vi "pulse_detector_usrp_implemented.vi"() -> ()   [LabVIEW 2021]
doc: "Acquires data from the Rx ports and streams the data to the host while receiving data from the host and generating the resulting waveform at the Tx ports of the NI USRP-294x/295x device. Use this VI as a template for the Simple NI-USRP Streaming sample project."
uses:
  <instrlib>/_niInstr/Register Bus/v1/FPGA/Public/Read Cmd Data.ctl
  SubVIs/Tx Parameters.ctl
  Host/SubVIs/Start Trigger.ctl
  SubVIs/DUC Parameters.ctl
  <instrlib>/_niInstr/DSP/v1/Shared/Public/IQ Impairments.ctl
  <instrlib>/_niInstr/DSP/v1/Shared/Public/IQ Gain.ctl
  SubVIs/Stream Control State.ctl
  SubVIs/Rx Parameters.ctl
  SubVIs/DDC Parameters.ctl
  reciver params.ctl
  <vilib>/Platform/TimedLoop/XDataNode/timing_clust.ctl
  <vilib>/Platform/TimedLoop/XDataNode/nitl_modes.ctl
  <vilib>/Platform/TimedLoop/XDataNode/wakeup.ctl
  <vilib>/rvi/Emulation/niFpgaSctlEmulationGetInTimedLoop.vi
  <vilib>/rvi/Emulation/niFpgaEmulationReportErrorSimple.vi
  <vilib>/rvi/Emulation/niFpgaGetClockAttributes.vi
  <vilib>/rvi/Emulation/niFpgaCriticalErrorInLSC.vi
  <vilib>/rvi/Emulation/niFpgaProcessEmulError.vi
  <vilib>/rvi/eio/common/nirviEmuTemplateMethod_errors.vi
  <vilib>/rvi/interface/RandomDataEmulation/niFpgaRandomDataHandleErrors.vi
  <vilib>/Platform/TimedLoop/XDataNode/XDataNode.xnode
  <vilib>/eio/EIONode/EIONode.xnode
  <vilib>/rvi/DataTransferAndStorage/Container/XNode/niFpgaContainer.xnode
  <vilib>/rvi/interface/RandomDataEmulation/nirviRandomDataFpgaReadWriteTemplate.vi
  <vilib>/Platform/TimedLoop/XDataNode/XDNodeRunTimeDep.lvlib
  <instrlib>/_niInstr/Register Bus/v1/FPGA/niInstr Register Bus v1 FPGA.lvlib
  <instrlib>/niUsrpRio/Config/v1/FPGA/niUsrpRio Config v1 FPGA.lvlib
  <instrlib>/_niInstr/DSP/v1/Shared/niInstr DSP v1 Shared.lvlib
panel:
  in  "reciver_params":T1
  in  "rx 3.led":T2(ring)
  in  "rx 2.led":T2(ring)
  in  "rx 0.led":T2(ring)
  in  "rx 1.led":T2(ring)
  in  "tx 0.led":enum16{"None", "RF 0/TX 1", "RF 1/TX 1"}(ring)
  in  "tx 1.led":enum16{"None", "RF 0/TX 1", "RF 1/TX 1"}(ring)
  in  "rx 3.stream enable":bool
  in  "rx 2.stream enable":bool
  out "rx 3.number of iq data overflows":u64
  out "rx 2.number of iq data overflows":u64
  in  "rx 3.phase":fxp<+/-,21,0>
  in  "rx 3.frequency shift":fxp<+/-,48,0> format="%#.48g"
  in  "rx 3.impairments":T3={"inline gain I"=0.9999923706054688, "inline gain Q"=0.9999923706054688, "cross gain I"=0.0, "cross gain Q"=0.0, "pre-gain offset I"=0.0, "pre-gain offset Q"=0.0, "post-gain offset I"=0.0, "post-gain offset Q"=0.0}
  in  "rx 2.phase":fxp<+/-,21,0>
  in  "rx 2.frequency shift":fxp<+/-,48,0> format="%#.48g"
  in  "rx 2.impairments":T3={"inline gain I"=0.9999923706054688, "inline gain Q"=0.9999923706054688, "cross gain I"=0.0, "cross gain Q"=0.0, "pre-gain offset I"=0.0, "pre-gain offset Q"=0.0, "post-gain offset I"=0.0, "post-gain offset Q"=0.0}
  out "tx.status":T5={"tx.state"=enum."Idle", "tx.samples processed"=0, "tx.number of fifo underflows"=0, "tx.number of iq data overflows"=[0, 0], "tx.dsp reset done"=FALSE}
  out "rx.status":T6={"rx.state"=enum."Idle", "rx.samples processed"=0, "rx.number of fifo overflows"=0, "rx.number of iq data overflows"=[0, 0], "rx.dsp reset done"=FALSE}
  in  "rx.output sample rate":fxp<+,48,1>
  in  "rx.delay":fxp<+/-,16,0>
  in  "rx 0.frequency shift":fxp<+/-,48,0> format="%#.48g"
  in  "rx 0.phase":fxp<+/-,21,0>
  in  "rx 0.impairments":T3={"inline gain I"=0.9999923706054688, "inline gain Q"=0.9999923706054688, "cross gain I"=0.0, "cross gain Q"=0.0, "pre-gain offset I"=0.0, "pre-gain offset Q"=0.0, "post-gain offset I"=0.0, "post-gain offset Q"=0.0}
  in  "rx 1.impairments":T3={"inline gain I"=0.9999923706054688, "inline gain Q"=0.9999923706054688, "cross gain I"=0.0, "cross gain Q"=0.0, "pre-gain offset I"=0.0, "pre-gain offset Q"=0.0, "post-gain offset I"=0.0, "post-gain offset Q"=0.0}
  in  "rx 1.frequency shift":fxp<+/-,48,0> format="%#.48g"
  in  "rx 1.phase":fxp<+/-,21,0>
  in  "tx.input sample rate":fxp<+,48,1>
  in  "tx.delay":fxp<+/-,18,0>
  in  "tx 0.frequency shift":fxp<+/-,48,0> format="%#.48g"
  in  "tx 0.phase":fxp<+/-,21,0>
  in  "tx 0.impairments":T3={"inline gain I"=0.9999923706054688, "inline gain Q"=0.9999923706054688, "cross gain I"=0.0, "cross gain Q"=0.0, "pre-gain offset I"=0.0, "pre-gain offset Q"=0.0, "post-gain offset I"=0.0, "post-gain offset Q"=0.0}
  in  "tx 0.gain":T7={"gain I"=1.0, "gain Q"=1.0}
  in  "tx 1.impairments":T3={"inline gain I"=0.9999923706054688, "inline gain Q"=0.9999923706054688, "cross gain I"=0.0, "cross gain Q"=0.0, "pre-gain offset I"=0.0, "pre-gain offset Q"=0.0, "post-gain offset I"=0.0, "post-gain offset Q"=0.0}
  in  "tx 1.frequency shift":fxp<+/-,48,0> format="%#.48g"
  in  "tx 1.phase":fxp<+/-,21,0>
  in  "tx 1.gain":T7={"gain I"=1.0, "gain Q"=1.0}
  in  "rx.reset":bool=TRUE
  in  "rx.samples to acquire":u32
  in  "rx.abort":bool
  in  "tx.abort":bool
  in  "tx.reset":bool=TRUE
  in  "tx.samples to generate":u32
  in  "rx 0.stream enable":bool
  in  "rx 1.stream enable":bool
  in  "rx.trigger select":T8=enum."Immediate"
  in  "rx.software trigger":bool
  in  "rx.trigger enable":bool
  in  "tx 0.stream enable":bool
  in  "tx 1.stream enable":bool
  in  "tx.trigger select":T8=enum."Immediate"
  in  "tx.software trigger":bool
  in  "tx.trigger enable":bool
  out "rx.parameters":T9={"rx.trigger select"=enum."Software", "rx.trigger enable"=FALSE, "rx.trigger sync enable"=FALSE, "rx.stream enable"=[FALSE, FALSE, FALSE, FALSE], "rx.software trigger"=FALSE, "rx.reset"=FALSE, "rx.abort"=FALSE, "rx.samples to acquire"=0, "rx.data sink"=enum."SFP Port 0", "rx.ddc parameters"=[{"output sample rate"=0.0, "delay"=0.0, "frequency shift"=0.0, "impairments"={"inline gain I"=0.0, "inline gain Q"=0.0, "cross gain I"=0.0, "cross gain Q"=0.0, "pre-gain offset I"=0.0, "pre-gain offset Q"=0.0, "post-gain offset I"=0.0, "post-gain offset Q"=0.0}, "phase"=0.0}, {"output sample rate"=0.0, "delay"=0.0, "frequency shift"=0.0, "impairments"={"inline gain I"=0.0, "inline gain Q"=0.0, "cross gain I"=0.0, "cross gain Q"=0.0, "pre-gain offset I"=0.0, "pre-gain offset Q"=0.0, "post-gain offset I"=0.0, "post-gain offset Q"=0.0}, "phase"=0.0}, {"output sample rate"=0.0, "delay"=0.0, "frequency shift"=0.0, "impairments"={"inline gain I"=0.0, "inline gain Q"=0.0, "cross gain I"=0.0, "cross gain Q"=0.0, "pre-gain offset I"=0.0, "pre-gain offset Q"=0.0, "post-gain offset I"=0.0, "post-gain offset Q"=0.0}, "phase"=0.0}, {"output sample rate"=0.0, "delay"=0.0, "frequency shift"=0.0, "impairments"={"inline gain I"=0.0, "inline gain Q"=0.0, "cross gain I"=0.0, "cross gain Q"=0.0, "pre-gain offset I"=0.0, "pre-gain offset Q"=0.0, "post-gain offset I"=0.0, "post-gain offset Q"=0.0}, "phase"=0.0}]} {"rx.ddc parameters"."frequency shift" format="%#.48g"}
  out "rx.samples processed":u32
  out "rx.state":T4
  out "rx 0.number of iq data overflows":u64
  out "rx.number of fifo overflows":u32
  out "tx.samples processed":u32
  out "tx.number of fifo underflows":u32
  out "tx 0.number of iq data overflows":u64
  out "tx.state":T4
  out "rx.dsp reset done":bool
  out "tx.dsp reset done":bool
  out "tx 1.number of iq data overflows":u64
  out "rx 1.number of iq data overflows":u64
  out "tx.parameters":T11={"tx.trigger select"=enum."Software", "tx.trigger enable"=FALSE, "tx.trigger sync enable"=FALSE, "tx.stream enable"=[FALSE, FALSE], "tx.software trigger"=FALSE, "tx.reset"=FALSE, "tx.abort"=FALSE, "tx.samples to generate"=0, "tx.data source"=enum."SFP Port 0", "tx.duc parameters"=[{"frequency shift"=0.0, "impairments"={"inline gain I"=0.0, "inline gain Q"=0.0, "cross gain I"=0.0, "cross gain Q"=0.0, "pre-gain offset I"=0.0, "pre-gain offset Q"=0.0, "post-gain offset I"=0.0, "post-gain offset Q"=0.0}, "phase"=0.0, "input sample rate"=0.0, "gain"={"gain I"=0.0, "gain Q"=0.0}, "delay"=0.0}, {"frequency shift"=0.0, "impairments"={"inline gain I"=0.0, "inline gain Q"=0.0, "cross gain I"=0.0, "cross gain Q"=0.0, "pre-gain offset I"=0.0, "pre-gain offset Q"=0.0, "post-gain offset I"=0.0, "post-gain offset Q"=0.0}, "phase"=0.0, "input sample rate"=0.0, "gain"={"gain I"=0.0, "gain Q"=0.0}, "delay"=0.0}]} {"tx.duc parameters"."frequency shift" format="%#.48g"}
  in  "rx.trigger sync enable":bool
  in  "tx.trigger sync enable":bool
  in  "rx.data sink":enum16{"SFP Port 0", "SFP Port 1", "Host"}(ring)=enum."Host"
  in  "tx.data source":enum16{"SFP Port 0", "SFP Port 1", "Host"}(ring)=enum."Host"
  in  "RF 1/Tx/Enable":bool
  in  "RF 1/Rx/Enable":bool
  in  "RF 0/Tx/Enable":bool
  in  "RF 0/Rx/Enable":bool
  in  "reg.host read.go rcvd 0":bool
  out "reg.notify host.go 0":bool
  in  "reg.notify host.go rcvd 0":bool
  out "reg.host read.data 0":T13
  in  "reg.reset 0":bool
  # "FPGA utilization for 120 MS/s"
  # "FPGA utilization for 200 MS/s"
  # "USRP RIO Simple Streaming FPGA"
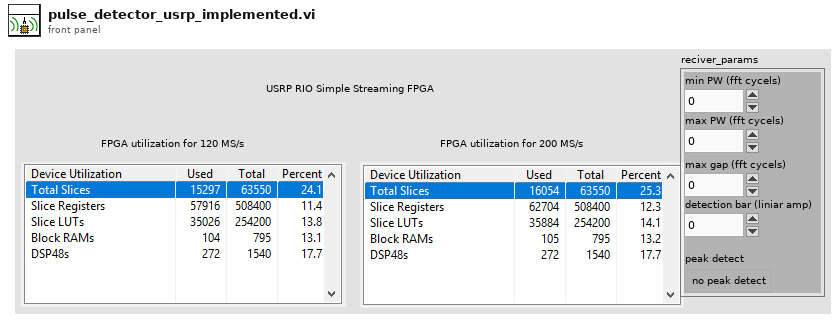
[diagram p1: front panel]
types:
  T1 = typedef "reciver params.ctl" = cluster{"min PW (fft cycels)":u16, "max PW (fft cycels)":u16, "max gap (fft cycels)":u8, "detection bar (liniar amp)":fxp<+,64,63>, "peak detect":bool}
  T2 = enum16{"None", "RF 0/RX 1", "RF 0/RX 2", "RF 1/RX 1", "RF 1/RX 2"}
  T3 = typedef "niInstr DSP v1 Shared.lvlib/IQ Impairments.ctl" = cluster{"inline gain I":fxp<+/-,18,1>, "inline gain Q":fxp<+/-,18,1>, "cross gain I":fxp<+/-,18,1>, "cross gain Q":fxp<+/-,18,1>, "pre-gain offset I":fxp<+/-,18,1>, "pre-gain offset Q":fxp<+/-,18,1>, "post-gain offset I":fxp<+/-,18,1>, "post-gain offset Q":fxp<+/-,18,1>}
  T4 = typedef "Stream Control State.ctl" = enum16{"Idle", "Active"}
  T5 = cluster{"tx.state":T4, "tx.samples processed":u32, "tx.number of fifo underflows":u32, "tx.number of iq data overflows":u64[], "tx.dsp reset done":bool}
  T6 = cluster{"rx.state":T4, "rx.samples processed":u32, "rx.number of fifo overflows":u32, "rx.number of iq data overflows":u64[], "rx.dsp reset done":bool}
  T7 = typedef "niInstr DSP v1 Shared.lvlib/IQ Gain.ctl" = cluster{"gain I":fxp<+/-,24,3>, "gain Q":fxp<+/-,24,3>}
  T8 = typedef "Start Trigger.ctl" = enum8{"Software", "Digital Edge", "Rx Start Trigger", "Tx Start Trigger", "Immediate", "Future Time Event"}
  T9 = typedef "Rx Parameters.ctl" = cluster{"rx.trigger select":T8, "rx.trigger enable":bool, "rx.trigger sync enable":bool, "rx.stream enable":bool[], "rx.software trigger":bool, "rx.reset":bool, "rx.abort":bool, "rx.samples to acquire":u32, "rx.data sink":enum16{"SFP Port 0", "SFP Port 1", "Host"}, "rx.ddc parameters":T10[]}
  T10 = typedef "DDC Parameters.ctl" = cluster{"output sample rate":fxp<+,48,1>, "delay":fxp<+/-,16,0>, "frequency shift":fxp<+/-,48,0>, "impairments":T3, "phase":fxp<+/-,21,0>}
  T11 = typedef "Tx Parameters.ctl" = cluster{"tx.trigger select":T8, "tx.trigger enable":bool, "tx.trigger sync enable":bool, "tx.stream enable":bool[], "tx.software trigger":bool, "tx.reset":bool, "tx.abort":bool, "tx.samples to generate":u32, "tx.data source":enum16{"SFP Port 0", "SFP Port 1", "Host"}, "tx.duc parameters":T12[]}
  T12 = typedef "DUC Parameters.ctl" = cluster{"frequency shift":fxp<+/-,48,0>, "impairments":T3, "phase":fxp<+/-,21,0>, "input sample rate":fxp<+,48,1>, "gain":T7, "delay":fxp<+/-,18,0>}
  T13 = typedef "niInstr Register Bus v1 FPGA.lvlib/Read Cmd Data.ctl" = cluster{"go":bool, "data":u32}
  T14 = typedef "XDNodeRunTimeDep.lvlib/timing_clust.ctl" = cluster{"Expected End [f-1]":u64, "Actual End [f-1]":u64, "Finished Late? [f-1]":bool, "Expected End [i-1]":u64, "Actual End [i-1]":u64, "Finished Late? [i-1]":bool, "Expected Start [i]":u64, "Actual Start [i]":u64, "Expected Start [f]":u64, "Actual Start [f]":u64, "Source Name":string, "Structure Name":string, "Period":i64, "Deadline":i64, "Offset":i64, "Start":i64, "Priority":i32, "Timeout":i32, "Mode":T15, "Wakeup Reason":T16, "Error":errorcluster, "Source Type":string, "Secondary Source Type":string, "Global End Time":u64, "Global Start Time":u64, "Frame Duration":u64, "Iteration Duration":u64, "Assigned CPU":i32, "I/O Scan Engine Mode":u32}
  T15 = typedef "XDNodeRunTimeDep.lvlib/nitl_modes.ctl" = enum32{"No Change", "Process missed periods, maintain original phase", "Discard missed periods, maintain original phase", "Process missed periods, ignore original phase", "Discard missed periods, ignore original phase"}
  T16 = typedef "XDNodeRunTimeDep.lvlib/wakeup.ctl" = enum32{"Normal", "Aborted", "Asynchronous wakeup", "Timing source error", "Timed loop error", "Timeout"}
  T17 = cluster{"tx 0.led":enum16{"None", "RF 0/TX 1", "RF 1/TX 1"}, "tx 1.led ":enum16{"None", "RF 0/TX 1", "RF 1/TX 1"}}
  T18 = cluster{"rx 0.led":enum16{"None", "RF 0/RX 1", "RF 0/RX 2", "RF 1/RX 1", "RF 1/RX 2"}, "rx 1.led":enum16{"None", "RF 0/RX 1", "RF 0/RX 2", "RF 1/RX 1", "RF 1/RX 2"}}
  T19 = cluster{"rx.trigger select":T8, "rx.trigger enable":bool, "rx.trigger sync enable":bool, bool[], "rx.software trigger":bool, "rx.reset":bool, "rx.abort":bool, "rx.samples to acquire":u32, "rx.data sink":enum16{"SFP Port 0", "SFP Port 1", "Host"}, T10[]}
  T20 = cluster{"tx.trigger select":T8, "tx.trigger enable":bool, "tx.trigger sync enable":bool, bool[], "tx.software trigger":bool, "tx.reset":bool, "tx.abort":bool, "tx.samples to generate":u32, "tx.data source":enum16{"SFP Port 0", "SFP Port 1", "Host"}, T12[]}
  T21 = cluster{"DAC FIFO Reset":refnum<k21>, "RF 0 Rx Swap IQ":refnum<k21>, "RF 0 Rx Negate I":refnum<k21>, "RF 0 Rx Negate Q":refnum<k21>, "RF 0 Rx Data Valid":refnum<k21>, "RF 0 Rx Data Ever Invalid":refnum<k21>, "clear RF 0 Rx Data Ever Invalid":refnum<k21>, "RF 0 Tx Swap IQ":refnum<k21>, "RF 0 Tx Negate I":refnum<k21>, "RF 0 Tx Negate Q":refnum<k21>, "RF 1 Rx Swap IQ":refnum<k21>, "RF 1 Rx Negate I":refnum<k21>, "RF 1 Rx Negate Q":refnum<k21>, "RF 1 Rx Data Valid":refnum<k21>, "RF 1 Rx Data Ever Invalid":refnum<k21>, "clear RF 1 Rx Data Ever Invalid":refnum<k21>, "RF 1 Tx Swap IQ":refnum<k21>, "RF 1 Tx Negate I":refnum<k21>, "RF 1 Tx Negate Q":refnum<k21>}
  T22 = typedef "niUsrpRio Synchronization v1 FPGA.lvlib/Resources.ctl" = cluster{"master":refnum<k21>, "meas.enable":refnum<k21>, "meas.ready":refnum<k21>, "meas.reset":refnum<k21>, "meas.arm":refnum<k21>, "meas.valid":refnum<k21>, "meas.value":refnum<k21>, "meas.oversample factor":refnum<k21>, "cptr":refnum<k21>, "cptr.adjust":refnum<k21>, "cptr.period":refnum<k21>}
  T23 = typedef "niUsrpRio Time v1 FPGA.lvlib/Time Resources.ctl" = cluster{"reset":refnum<k21>, "time":refnum<k21>, "time.previous cptr":refnum<k21>, "new time":refnum<k21>, "new time.when":refnum<k21>, "new time.set":refnum<k21>, "which edge of ref":refnum<k21>, "pps source":refnum<k21>, "internal pps period":refnum<k21>}
  T24 = typedef "niUsrpRio Time v1 FPGA.lvlib/Future Event Resources.ctl" = cluster{"reset":refnum<k21>, "future event.time":refnum<k21>, "future event.ready":refnum<k21>, "future event.set":refnum<k21>, "future event.clear":refnum<k21>, "future event.set in past":refnum<k21>}
  T25 = cluster{"time.resources":T23, "future event.resources":T24, "future event.resources":T24, "future event.resources":T24}
  T26 = typedef "niInstr Register Bus v1 FPGA.lvlib/Register Instruction.ctl" = cluster{"subsystem":u8, "address":u16, "data":u32, "valid":bool, "read":bool}
  T27 = typedef "niInstr Register Bus v1 FPGA.lvlib/Read Completion.ctl" = cluster{"data":u32, "valid":bool}
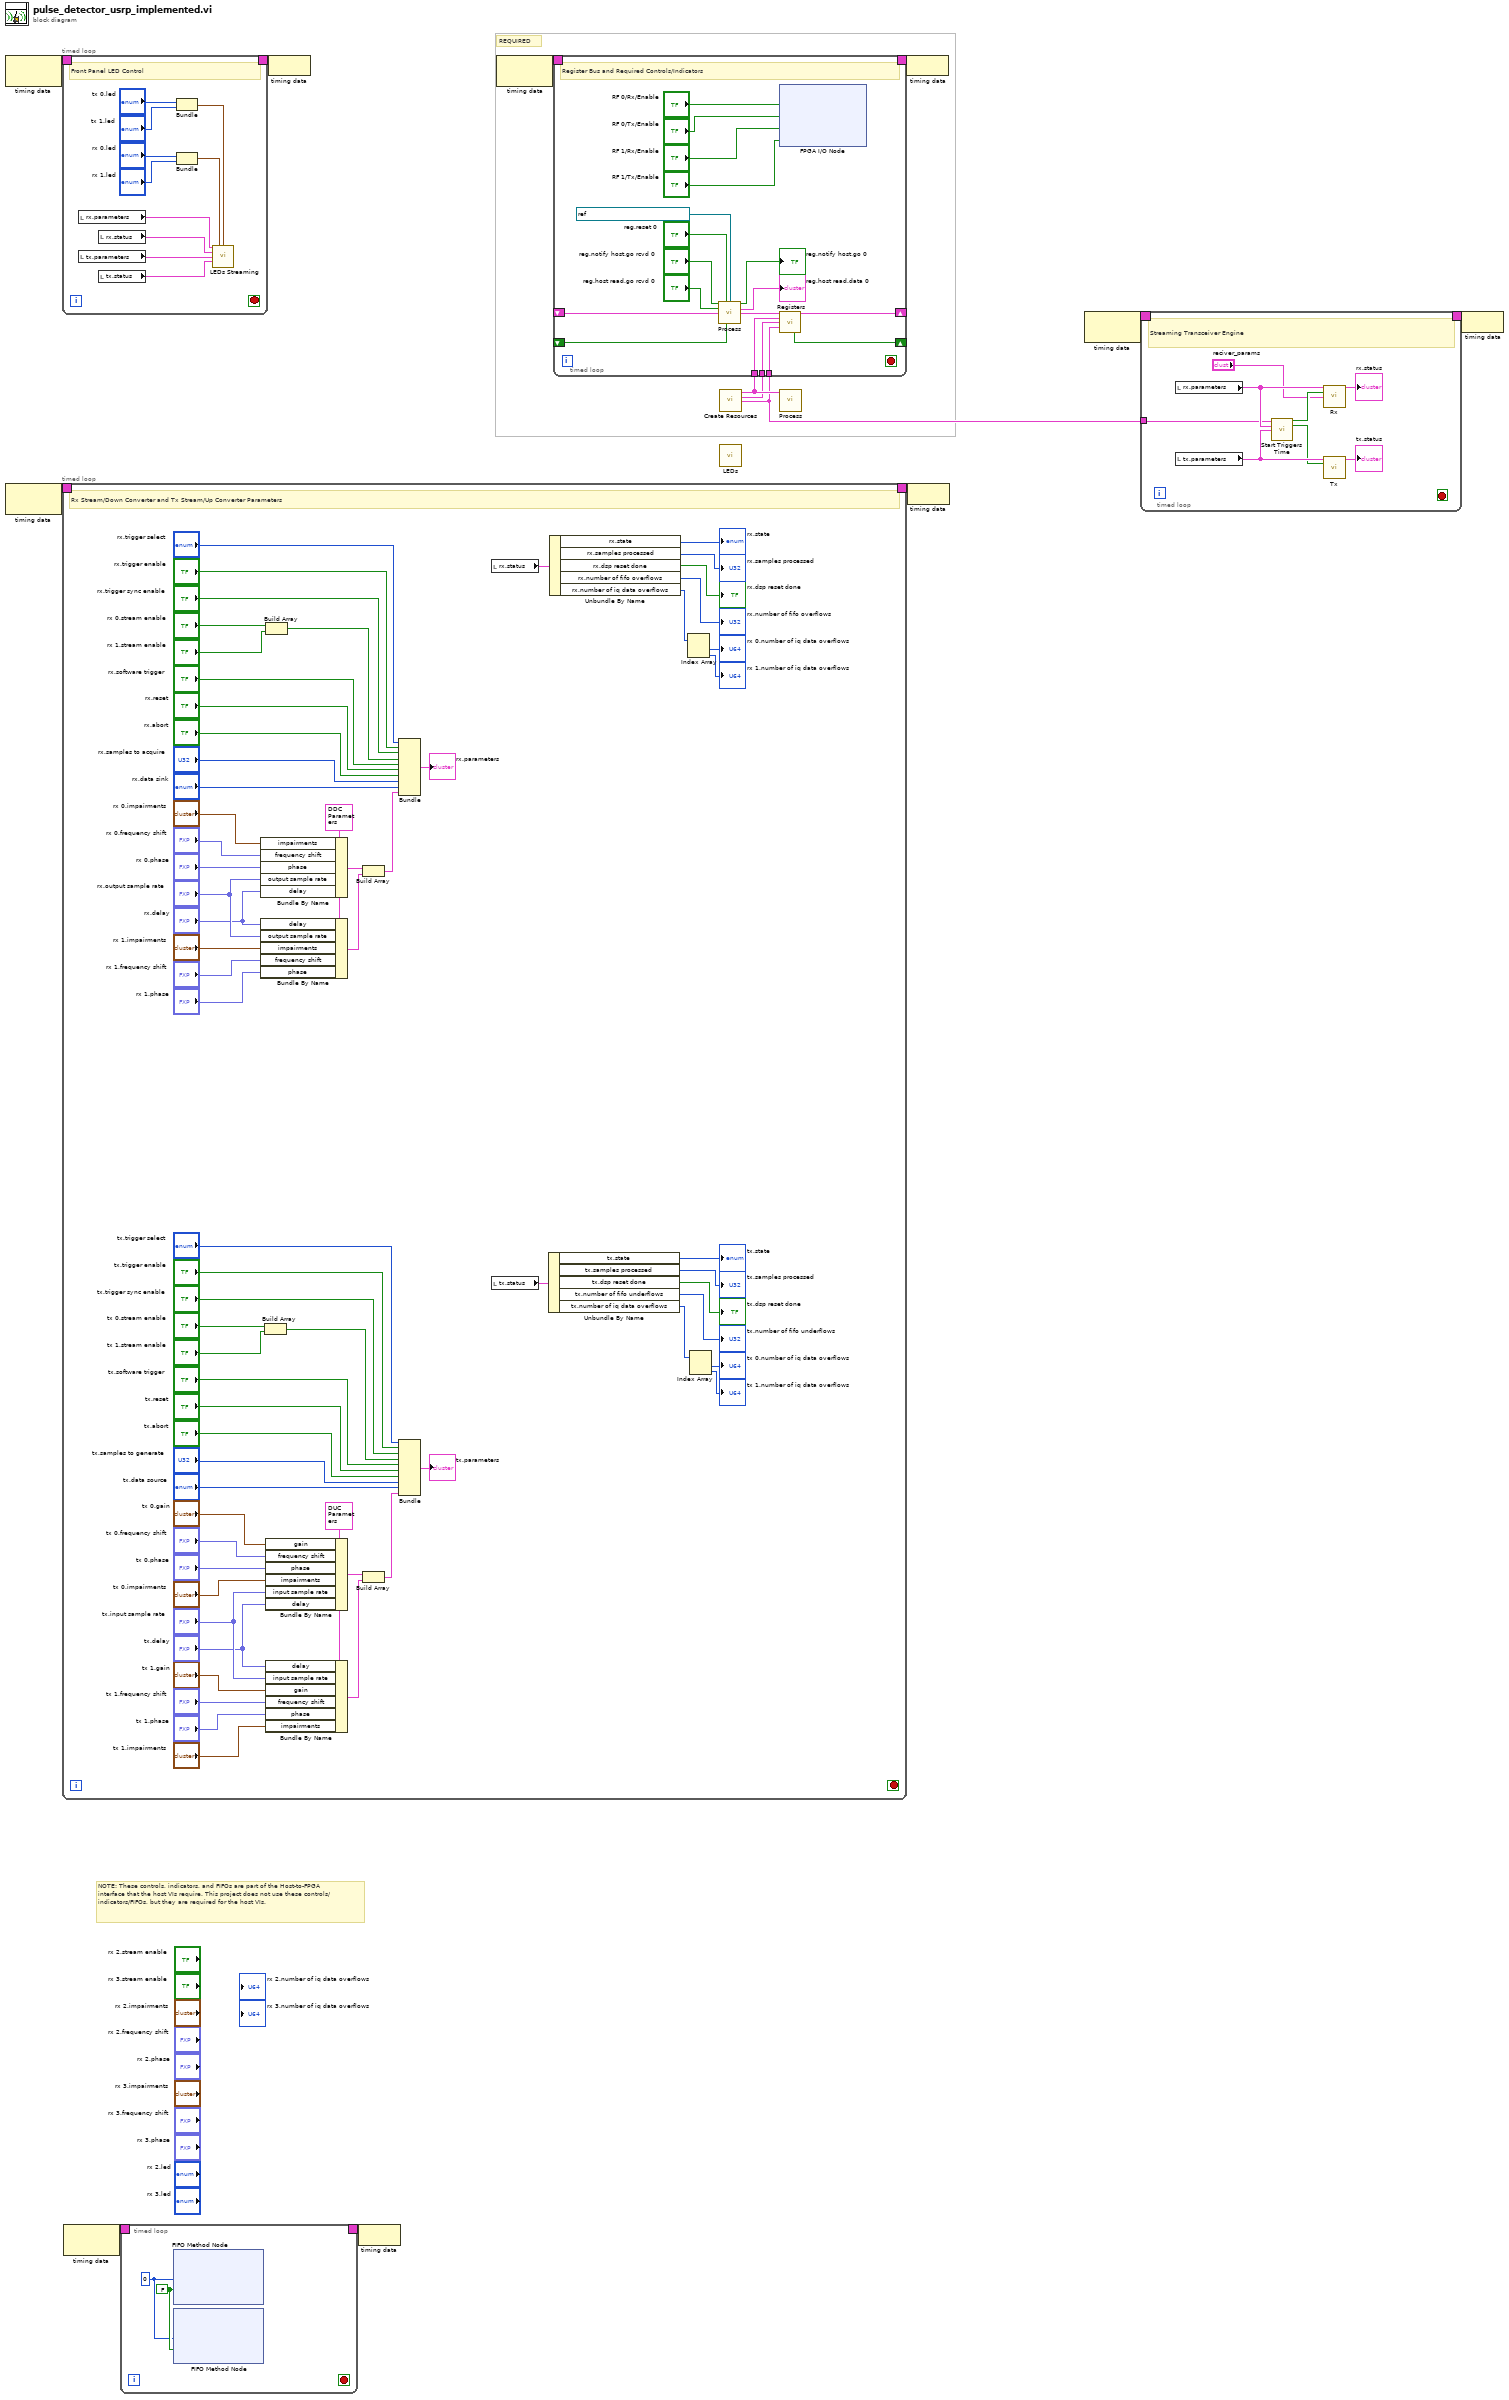
[diagram p0: block diagram]
diagram:
  # "NOTE: These controls, indicators, and FIFOs are part of the Host-to-FPGA interface that the host VIs require. This project does not use these controls/indicators/FIFOs, but they are required for the host VIs."
  # "REQUIRED"
  n1 = node-c288() -> (w2:T14)  [unwired: 1 in]
  n2 = node-c288() -> (w9:T14)  [unwired: 1 in]
  n3 = timed-loop {
    timing: w2 -> [_]
    timing-out: [_] -> w1
    stop <- _ stop-if-true
    # "Front Panel LED Control"
    n4 = local read "rx.parameters"() -> (w17:T9)
    n5 = local read "tx.parameters"() -> (w15:T11)
    n6 = local read "rx.status"() -> (w16:T6)
    n7 = local read "tx.status"() -> (w14:T5)
    n8 = Bundle("tx 0.led"="tx 0.led", "tx 1.led"="tx 1.led") -> (w18:T17)  [unwired: 1 in]
    n9 = Bundle("rx 0.led"="rx 0.led", "rx 1.led"="rx 1.led") -> (w19:T18)  [unwired: 1 in]
    n10 = call "LEDs Streaming.vi"("rx.parameters"=w17, "rx.leds"=w19, "tx.leds"=w18, "rx.status"=w16, "tx.parameters"=w15, "tx.status"=w14) -> ()  [unwired: 10 in]
  }
  n11 = timed-loop {
    timing: w9 -> [_]
    timing-out: [_] -> w8
    stop <- _ stop-if-true
    w80 = T12 {"frequency shift"=0.0, "impairments"={"inline gain I"=0.9999923706054688, "inline gain Q"=0.9999923706054688, "cross gain I"=0.0, "cross gain Q"=0.0, "pre-gain offset I"=0.0, "pre-gain offset Q"=0.0, "post-gain offset I"=0.0, "post-gain offset Q"=0.0}, "phase"=0.0, "input sample rate"=0.0, "gain"={"gain I"=1.0, "gain Q"=1.0}, "delay"=0.0} ("DUC Parameters")
    w91 = T10 {"output sample rate"=1.0, "delay"=0.0, "frequency shift"=0.0, "impairments"={"inline gain I"=0.9999923706054688, "inline gain Q"=0.9999923706054688, "cross gain I"=0.0, "cross gain Q"=0.0, "pre-gain offset I"=0.0, "pre-gain offset Q"=0.0, "post-gain offset I"=0.0, "post-gain offset Q"=0.0}, "phase"=0.0} ("DDC Parameters")
    # "Rx Stream/Down Converter and Tx Stream/Up Converter Parameters"
    n12 = Bundle By Name(cluster=w91, "impairments"="rx 0.impairments", "frequency shift"="rx 0.frequency shift", "phase"="rx 0.phase", "output sample rate"="rx.output sample rate", "delay"="rx.delay") -> (w89:T10)
    n13 = Bundle By Name(cluster=w91, "delay"="rx.delay", "output sample rate"="rx.output sample rate", "impairments"="rx 1.impairments", "frequency shift"="rx 1.frequency shift", "phase"="rx 1.phase") -> (w90:T10)
    n14 = Build Array("tx 0.stream enable", "tx 1.stream enable") -> (w37:bool[])
    n15 = Build Array("rx 0.stream enable", "rx 1.stream enable") -> (w39:bool[])
    n16 = Bundle By Name(cluster=w80, "gain"="tx 0.gain", "frequency shift"="tx 0.frequency shift", "phase"="tx 0.phase", "impairments"="tx 0.impairments", "input sample rate"="tx.input sample rate", "delay"="tx.delay") -> (w78:T12)
    n17 = Bundle By Name(cluster=w80, "delay"="tx.delay", "input sample rate"="tx.input sample rate", "gain"="tx 1.gain", "frequency shift"="tx 1.frequency shift", "phase"="tx 1.phase", "impairments"="tx 1.impairments") -> (w79:T12)
    n18 = Build Array(w89, w90) -> (w60:T10[])
    n19 = Build Array(w78, w79) -> (w58:T12[])
    n20 = Bundle("rx.trigger select"="rx.trigger select", "rx.trigger enable"="rx.trigger enable", "rx.trigger sync enable"="rx.trigger sync enable", w39, "rx.software trigger"="rx.software trigger", "rx.reset"="rx.reset", "rx.abort"="rx.abort", "rx.samples to acquire"="rx.samples to acquire", "rx.data sink"="rx.data sink", w60) -> (→"rx.parameters":T19)  [unwired: 1 in]
    n21 = Bundle("tx.trigger select"="tx.trigger select", "tx.trigger enable"="tx.trigger enable", "tx.trigger sync enable"="tx.trigger sync enable", w37, "tx.software trigger"="tx.software trigger", "tx.reset"="tx.reset", "tx.abort"="tx.abort", "tx.samples to generate"="tx.samples to generate", "tx.data source"="tx.data source", w58) -> (→"tx.parameters":T20)  [unwired: 1 in]
    n22 = local read "rx.status"() -> (w51:T6)
    n23 = local read "tx.status"() -> (w48:T5)
    n24 = Unbundle By Name(w48) -> ("tx.state"=→"tx.state":T4, "tx.samples processed"=→"tx.samples processed":u32, "tx.dsp reset done"=→"tx.dsp reset done":bool, "tx.number of fifo underflows"=→"tx.number of fifo underflows":u32, "tx.number of iq data overflows"=w31:u64[])
    n25 = Unbundle By Name(w51) -> ("rx.state"=→"rx.state":T4, "rx.samples processed"=→"rx.samples processed":u32, "rx.dsp reset done"=→"rx.dsp reset done":bool, "rx.number of fifo overflows"=→"rx.number of fifo overflows":u32, "rx.number of iq data overflows"=w28:u64[])
    n26 = Index Array(array=w28) -> (element #1=→"rx 0.number of iq data overflows":u64, element #2=→"rx 1.number of iq data overflows":u64)  [unwired: 2 in]
    n27 = Index Array(array=w31) -> (element #1=→"tx 0.number of iq data overflows":u64, element #2=→"tx 1.number of iq data overflows":u64)  [unwired: 2 in]
  }
  n28 = node-c288() -> (w4:T14)  [unwired: 1 in]
  n29 = timed-loop {
    timing: w4 -> [_]
    timing-out: [_] -> w3
    stop <- _ stop-if-true
    w94 = u32 0 ("Element")
    w95 = FALSE ("Input Valid")
    n30 = xnode ("FIFO Method Node")("Element"=w94, "Input Valid"=w95) -> ()  [unwired: 1 in, 2 out]
    n31 = xnode ("FIFO Method Node")("Element"=w94, "Input Valid"=w95) -> ()  [unwired: 1 in, 2 out]
  }
  n32 = node-c288(w1) -> ()
  n33 = node-c288(w3) -> ()
  n34 = node-c288() -> (w13:T14)  [unwired: 1 in]
  n35 = call "Create Resources.vi"() -> ("config.resources"=w7:T21, "sync.resources"=w6:T22, "time.resources"=w5:T25)  [unwired: 13 in]
  n36 = timed-loop "Register Bus and Required Controls/Indicators" {
    timing: w13 -> [_]
    timing-out: [_] -> w12
    shift-right: [w112] -> _
    shift-left: _ -> [w111]
    shift-right: [w106] -> _
    shift-left: _ -> [w110]
    tunnel: w7 -> [w104]
    tunnel: w6 -> [w103]
    tunnel: w5 -> [w102]
    stop <- _ stop-if-true
    # "Register Bus and Required Controls/Indicators"
    n37 = call <instrlib>:"Process.vi"("reg.notify host.go rcvd"="reg.notify host.go rcvd 0", "reg.reset"="reg.reset 0", "reg.host instruction fifo"=refnum<k21> "reg.host instruction fifo 0", "reg.host read.go rcvd"="reg.host read.go rcvd 0", "read completion"=w111, "ready for output"=w110) -> ("reg.notify host.go"=→"reg.notify host.go 0":bool, "reg.host read.data"=→"reg.host read.data 0":T13, "register instruction"=w105:T26)  [unwired: 7 in]
    n38 = xnode ("FPGA I/O Node")("RF 0/Rx/Enable"="RF 0/Rx/Enable", "RF 0/Tx/Enable"="RF 0/Tx/Enable", "RF 1/Rx/Enable"="RF 1/Rx/Enable", "RF 1/Tx/Enable"="RF 1/Tx/Enable") -> ()  [unwired: 4 in, 4 out]
    n39 = call "Registers.vi"("register instruction"=w105, "config.resources"=w104, "sync.resources"=w103, "time.resources"=w102) -> ("read completion out"=w112:T27, "ready for input"=w106:bool)  [unwired: 10 in]
  }
  n40 = call "LEDs.vi"() -> ()  [unwired: 1 in]
  n41 = call <instrlib>:"Process.vi"("resources"=w7) -> ()  [unwired: 15 in]
  n42 = node-c288(w12) -> ()
  n43 = node-c288(w8) -> ()
  n44 = node-c288() -> (w11:T14)  [unwired: 1 in]
  n45 = timed-loop "Streaming Transceiver Engine" {
    timing: w11 -> [_]
    timing-out: [_] -> w10
    tunnel: w5 -> [w119]
    stop <- _ stop-if-true
    # "Streaming Transceiver Engine"
    n46 = local read "rx.parameters"() -> (w123:T9)
    n47 = local read "tx.parameters"() -> (w124:T11)
    n48 = call "Start Triggers Time.vi"("time.resources"=w119, "rx.parameters"=w123, "tx.parameters"=w124) -> ("rx.start trigger"=w125:bool, "tx.start trigger"=w122:bool)  [unwired: 11 in]
    n49 = call "Rx.vi"("rx.parameters"=w123, "rx.start trigger"=w125, "reciver_params"="reciver_params") -> ("rx.status"=→"rx.status":T6)  [unwired: 12 in]
    n50 = call "Tx.vi"("tx.parameters"=w124, "tx.start trigger"=w122) -> ("tx.status"=→"tx.status":T5)  [unwired: 13 in]
  }
  n51 = node-c288(w10) -> ()
